vi "testStringNotIncluded.vi"() -> ()   [LabVIEW 2019, in "AssertionTest.lvlib" / "ErrorMessageContainsString.lvlib"]
uses:
  ErrorMessageContainsString.lvlib
  <vilib>/Utility/error.llb/Error Cluster From Error Code.vi
  <vilib>/ErrorRing/Error Ring.xnode
  Assertion/Assertion.lvlib
  AssertionTest.lvlib
  e8b37827-c40c-4938-b4cd-332d526e978e.vi
panel:
  out "error out":errorcluster
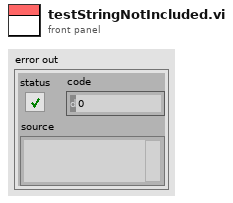
[diagram p1: front panel]
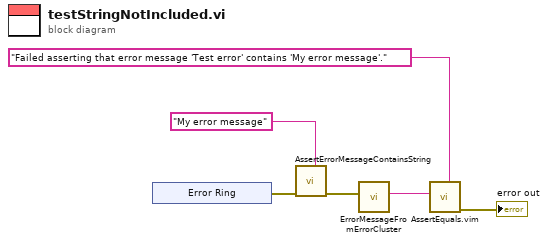
[diagram p0: block diagram]
diagram:
  n1 = xnode "Error Ring"() -> ("error out"=w3:errorcluster)
  n2 = call "AssertErrorMessageContainsString.vi"("Expected"="My error message", "error in (no error)"=w3) -> ("error out"=w2:errorcluster)  [unwired: 9 in]
  n3 = call "ErrorMessageFromErrorCluster.vi"("Error"=w2) -> ("Error Message"=w5:string)  [unwired: 10 in]
  n4 = call "AssertEquals.vim"("Expected"="Failed asserting that error message 'Test error' contains 'My error message'." ("Needle"), "Actual"=w5) -> ("error out"=→"error out":errorcluster)  [unwired: 9 in]
